vi "DataLogger.register trendmsg.vi"(8 "error in (no error)":errorcluster, 11 "i ref in":refnum<vi>) -> (0 "error out":errorcluster, 3 "i ref out":refnum<vi>)   [LabVIEW 2014, in "DataLogger.lvlib"]
uses:
  DataLogger.lvlib
  CS_Core/BaseProcess/BaseProcess.event definition.ctl
  CS_Core/CAEObj/CAEObj.event definition.ctl
  CS_Core/BaseProcess/BaseProcess.descriptor string definition.ctl
  CS_Core/BaseProcess/BaseProcess.lvlib
  CS_Core/CAEObj/CAEObj.lvlib
panel:
  in  "element":T1
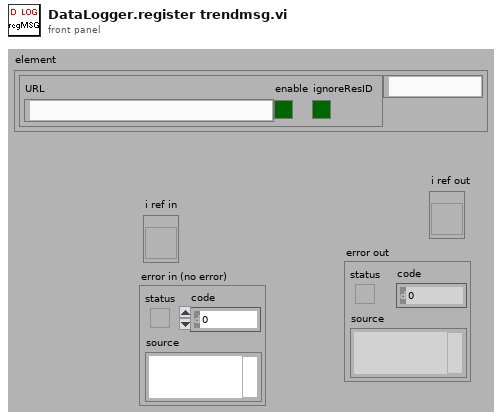
[diagram p1: front panel]
types:
  T1 = typedef "BaseProcess.lvlib/BaseProcess.event definition.ctl" = cluster{"CAEEvtDef":T2, "Data Descriptor":T3}
  T2 = typedef "CAEObj.lvlib/CAEObj.event definition.ctl" = cluster{"URL":string, "enable":bool, "ignoreResID":bool}
  T3 = typedef "BaseProcess.lvlib/BaseProcess.descriptor string definition.ctl" = string
  T4 = typedef "DataLogger.lvlib/DataLogger.i attribute.ctl" = cluster{"Service Names":string[], "Path":string[], "Service Alarm Index":i32[], "Service Alarm Limit1":dbl[], "Service Alarm Limit2":dbl[], "Service Alarm Indicator":bool[], "alarmID":i32, "pathID":i32, "SoundDeviceID":i32, "SoundFile":string, "SoundID":i32, "SoundFileID":i32}
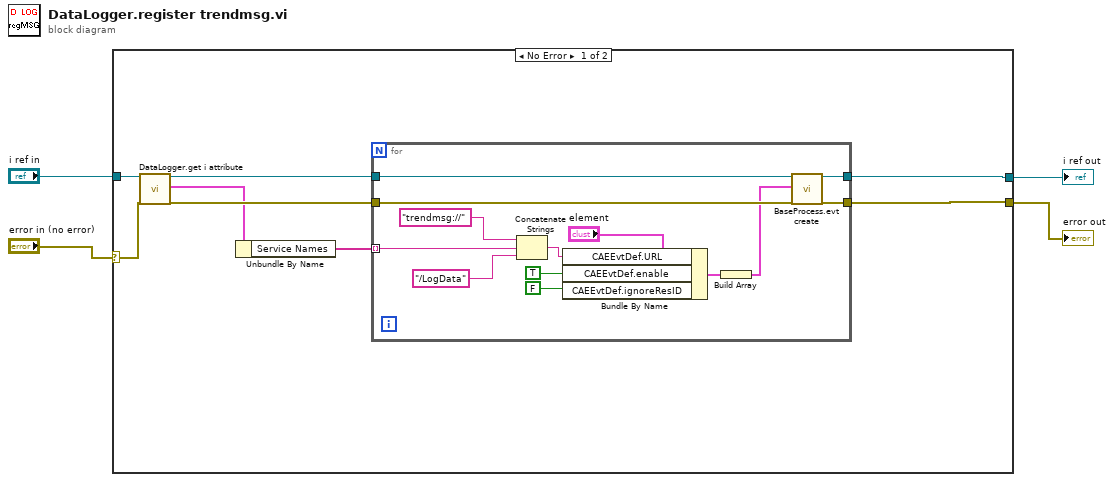
[diagram p0: block diagram]
diagram:
  n1 = case shown="No Error" "error in (no error)" {
    selector: "error in (no error)" -> [w8 w26]
    tunnel: "i ref in" -> [w9 w27]
    tunnel: [w7 w27] -> w2
    tunnel: [w6 w26] -> w1
    frame No Error {
      n2 = call "DataLogger.get i attribute.vi"("i ref in"=w9, "error in (no error)"=w8) -> ("i ref out"=w12:refnum<vi>, "i attribute"=w10:T4, "error out"=w11:errorcluster)  [unwired: 15 in]
      n3 = Unbundle By Name(w10) -> ("Service Names"=w5:string[])
      n4 = for {
        tunnel: w5 -> [w18] mode=indexing
        tunnel: w12 -> [w17]
        tunnel: w11 -> [w16]
        tunnel: [w15] -> w6
        tunnel: [w14] -> w7
        n5 = Concatenate Strings("trendmsg://" ("string"), w18, "/LogData" ("string")) -> (w22:string)
        n6 = Bundle By Name(cluster="element", "CAEEvtDef.URL"=w22, "CAEEvtDef.enable"=TRUE, "CAEEvtDef.ignoreResID"=FALSE) -> (w19:T1)
        n7 = Build Array(w19) -> (w13:T1[])
        n8 = call "BaseProcess.evt create.vi"("i ref in"=w17, "newEvents"=w13, "error in (no error)"=w16) -> ("i ref out"=w14:refnum<vi>, "error out"=w15:errorcluster)  [unwired: 13 in, 2 out]
      }
    }
    frame Error {
    }
  }
  "error out" <- w1
  "i ref out" <- w2
